vi "Return_Data.vi"(8 "error in (no error)":errorcluster caption="entrée d'erreur (pas d'erreur)", 11 "Class Instrument Firebase Altyor en entrée":refnum<class "Class Instrument Database Altyor.lvclass">) -> (0 "error out":errorcluster caption="sortie d'erreur", 2 "Data_Json":string, 3 "Class Instrument Firebase Altyor en sortie":refnum<class "Class Instrument Database Altyor.lvclass">)   [LabVIEW 2020, in "Library Instrument & Equipement.lvlib" / "Library Instruments.lvlib" / "Class Instrument Database Altyor.lvclass"]
uses:
  Class Instrument Database Altyor.lvclass
  Class Instrument Database Altyor.lvclass/Class Instrument Database Altyor.ctl
  JSON API/Variant JSON/Variant to JSON.vi
  JSON API/JSON Value/Get Item by name array.vi
  Database/Database Altyor/Database Altyor.lvclass
  JSON API/JSON Value/JSON Value.lvclass
  JSON API/Get Polymorphic/JSON GetSet.lvlib
  JSON API/Variant JSON/Variant JSON.lvlib
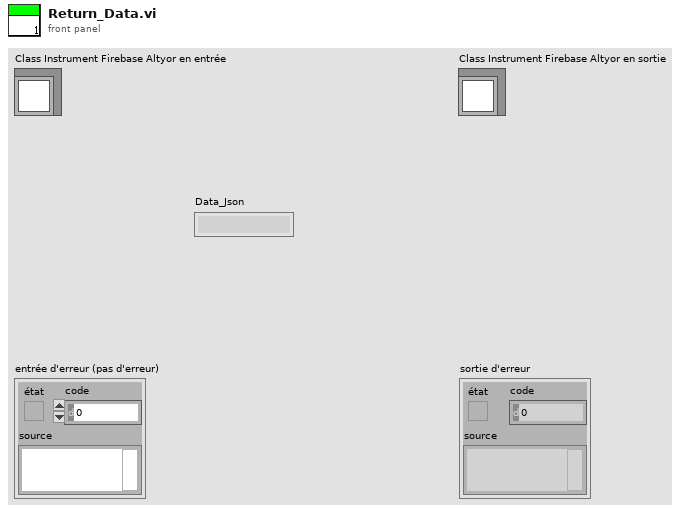
[diagram p1: front panel]
types:
  T1 = cluster{"idTest":u32, "CreationDate":string, "EndOfProduction":string, "OrderNumber":string, "Batch":string, "ProductName":string, "PartNumber":string, "SerialNumber":string, "Operator":string, "Result":string, "AdditionalInformation":string}[]
  T2 = cluster{"Key_Test":u32, "idTest":u32, "MainTest":string, "Name":string, "StartOfTest":string, "EndOfTest":string, "Result":string, "LimitMax":string, "Value":string, "LimitMin":string, "Type":string}[]
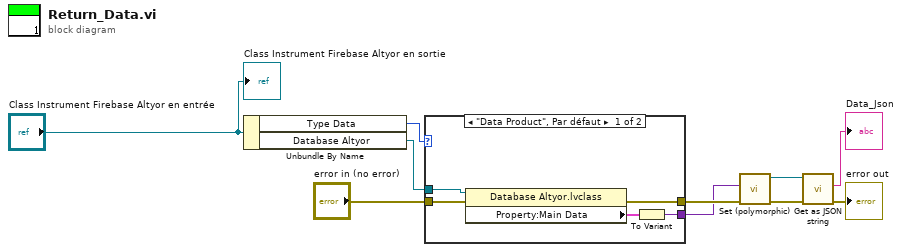
[diagram p0: block diagram]
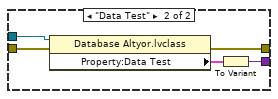
[diagram p2: hidden frame]
diagram:
  n1 = Unbundle By Name("Class Instrument Firebase Altyor en entrée") -> ("Type Data"=w10:enum16{"Data Product", "Data Test"}, "Database Altyor"=w8:refnum<class "Database Altyor.lvclass">)
  n2 = case shown="\"Data Product\", Par défaut" w10 {
    tunnel: w8 -> [w14 w20]
    tunnel: "error in (no error)" -> [w15 w19]
    tunnel: [w13 w18] -> w4
    tunnel: [w11 w16] -> w1
    frame "Data Product", Default {
      n3 = property class="Database Altyor.lvclass"(reference=w14, error in=w15) -> (error out=w13:errorcluster, "Property:Main Data"=w12:T1)  [unwired: 1 out]
      n4 = To Variant(anything=w12) -> (Variant=w11:variant)
    }
    frame "Data Test" {
      n5 = property class="Database Altyor.lvclass"(reference=w20, error in=w19) -> (error out=w18:errorcluster, "Property:Data Test"=w17:T2)  [unwired: 1 out]
      n6 = To Variant(anything=w17) -> (Variant=w16:variant)
    }
  }
  n7 = call-poly "Set (polymorphic).vi"("error in (no error)"=w4, "Variant"=w1) -> ("error out"=w5:errorcluster, "JSON Value out"=w6:refnum<class "JSON Value.lvclass">)  [unwired: 8 in]
  n8 = call "Get as JSON string.vi"("error in (no error)"=w5, "JSON Value in"=w6) -> ("error out"=→"error out":errorcluster, "<JSON>"=→"Data_Json":string)  [unwired: 8 in]
  "Class Instrument Firebase Altyor en sortie" <- "Class Instrument Firebase Altyor en entrée"
